vi "Image Calibration.vi"(0 "pObjectImage":u16, 1 "nMode":i32, 2 "bBackGround":i32, 5 "lpszRefPath":string, 7 "nWidth":i32, 9 "nHeight":i32, 11 "error in (no error)":errorcluster, 12 "rectMargin":cluster{"l":i32, "t":i32, "r":i32, "b":i32}) -> (4 "pObjectImage out":u16, 6 "lpszRefPath out":string, 8 "function return":i32, 15 "error out":errorcluster)   [LabVIEW 2017, in "imgCalibration.lvlib"]
doc: "DLLFunction int __stdcall ImageCalibration(unsigned short* pObjectImage, LPCTSTR lpszRefPath, int nWidth, int nHeight, int nMode, CRect rectMargin, BOOL bBackGround);"
uses:
  imgCalibration.lvlib
  lib/CalibrationDLL.dll
panel:
  out "rectMargin out":cluster{"l":i32, "t":i32, "r":i32, "b":i32}
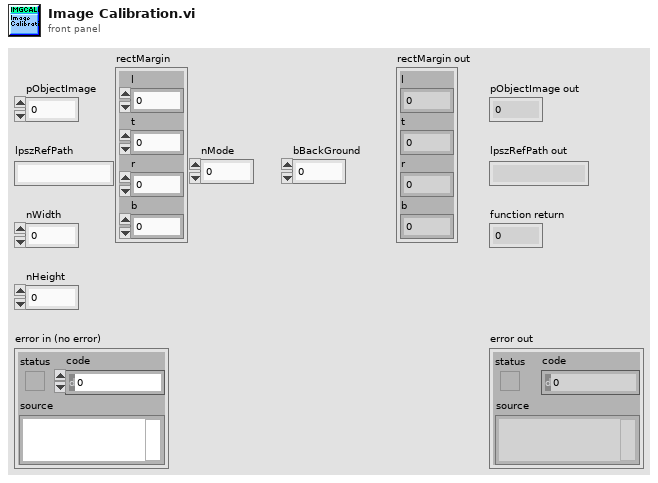
[diagram p1: front panel]
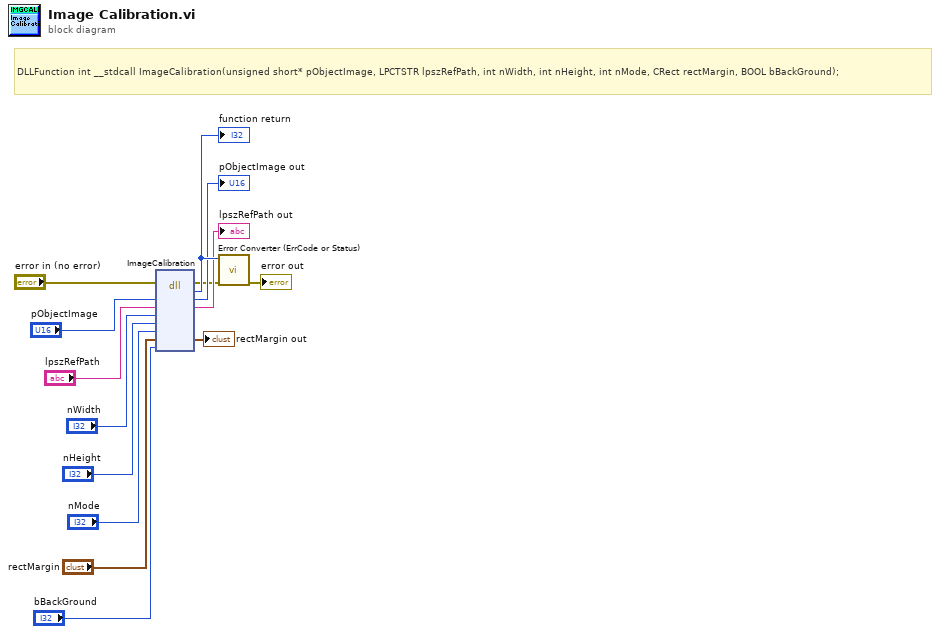
[diagram p0: block diagram]
diagram:
  # "DLLFunction int __stdcall ImageCalibration(unsigned short* pObjectImage, LPCTSTR lpszRefPath, int nWidth, int nHeight, int nMode, CRect rectMargin, BOOL bBackGround);"
  n1 = dll-call lib="F:/BonTechFlatPanelLVDriver/lib/CalibrationDLL.*" fn="ImageCalibration"(error in="error in (no error)", "pObjectImage"="pObjectImage", "lpszRefPath"="lpszRefPath", "nWidth"="nWidth", "nHeight"="nHeight", "nMode"="nMode", "rectMargin out"="rectMargin", "bBackGround"="bBackGround") -> (error out=w4:errorcluster, "return type"=w14:i32, "pObjectImage"=→"pObjectImage out":u16, "lpszRefPath"=→"lpszRefPath out":string, "rectMargin out"=→"rectMargin out":cluster{"l":i32, "t":i32, "r":i32, "b":i32})  [unwired: 6 in, 1 out]
  "function return" <- w14
  n2 = call "Error Converter (ErrCode or Status).vi"("error in (no error)"=w4, "error code"=w14) -> ("error out"=→"error out":errorcluster)  [unwired: 9 in]
